vi "Slope-Intercept.vi"(8 "Intercept":dbl, 9 "Slope":dbl, 10 "Value":dbl) -> (2 "Scaled Value":dbl)   [LabVIEW 2013, in "DAQmx(AI).lvclass"]
uses:
  DAQmx(AI).lvclass
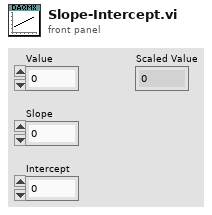
[diagram p1: front panel]
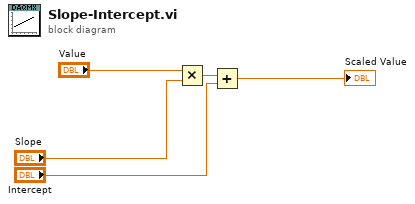
[diagram p0: block diagram]
diagram:
  n1 = Multiply(x="Value", y="Slope") -> (x*y=w2:dbl)
  n2 = Add(x=w2, y="Intercept") -> (x+y=→"Scaled Value":dbl)
